vi "Update Response.vi"(5 "Time":dbl format="%.2f", 7 "Devices in":T1[](array[typedef]), 8 "Last Updates in":dbl[](array[numeric]), 9 "MB response in":dbl[](array[numeric]), 10 "MB responses in":dbl[][](array[numeric]), 11 "MB ID-Address":T1) -> (0 "Last Updates out":dbl[](array[numeric]), 2 "MB responses out":dbl[][](array[numeric]))   [LabVIEW 2019]
uses:
  MB ID-Address.ctl
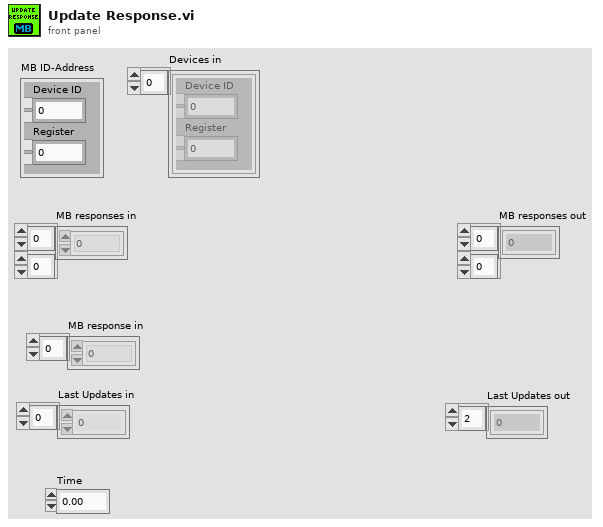
[diagram p1: front panel]
types:
  T1 = typedef "MB ID-Address.ctl" = cluster{"Device ID":u8, "Register":u16}
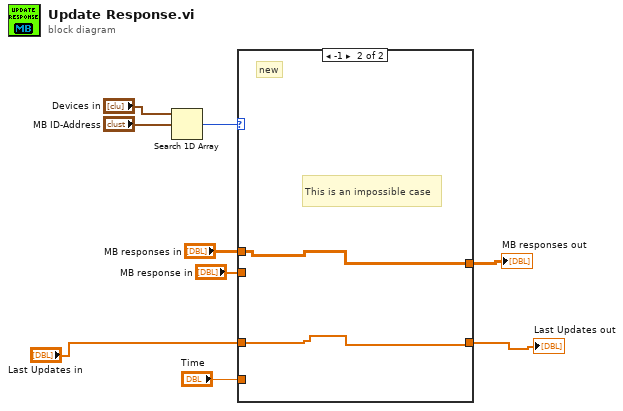
[diagram p0: block diagram]
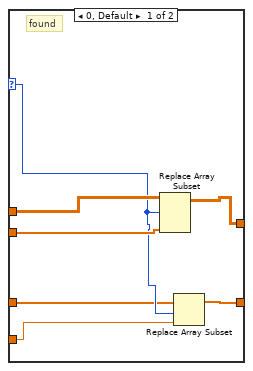
[diagram p2: hidden frame]
diagram:
  n1 = Search 1D Array(1D array="Devices in", element="MB ID-Address") -> (index of element=w9:i32)  [unwired: 1 in]
  n2 = case shown="-1" w9 {
    selector: w9 -> [w13 _]
    tunnel: "MB response in" -> [w14 _]
    tunnel: "MB responses in" -> [w15 w18]
    tunnel: [w16 w18] -> w6
    tunnel: "Last Updates in" -> [w12 w17]
    tunnel: [w11 w17] -> w5
    tunnel: "Time" -> [w10 _]
    frame 0, Default {
      # "found"
      n3 = Replace Array Subset(array=w15, new element=w14, index (row)=w13) -> (w16:dbl[][])  [unwired: 1 in]
      n4 = Replace Array Subset(array=w12, new element=w10, index=w13) -> (w11:dbl[])
    }
    frame -1 {
      # "This is an impossible case"
      # "new"
    }
  }
  "MB responses out" <- w6
  "Last Updates out" <- w5
